vi "IX83 Send Command.vi"(0 "Connection ID":refnum<k5>, 2 "Wait for Reply":bool=TRUE, 7 "Cmd":string, 11 "Error In":errorcluster) -> (4 "Connection ID Out":refnum<k5>, 8 "CMD Reply":string, 15 "Error Out":errorcluster)   [LabVIEW 2020]
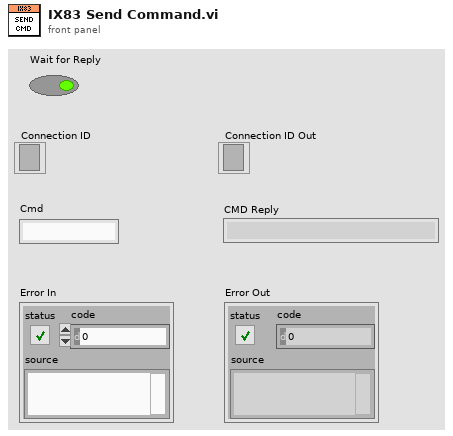
[diagram p1: front panel]
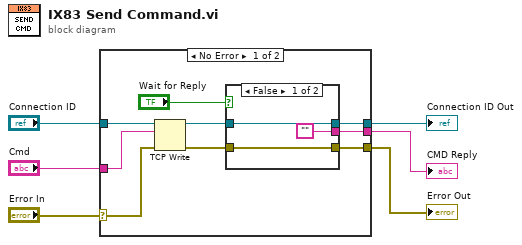
[diagram p0: block diagram]
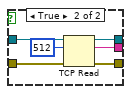
[diagram p2: hidden frame]
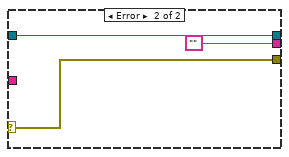
[diagram p3: hidden frame]
diagram:
  n1 = case shown="No Error" "Error In" {
    selector: "Error In" -> [w11 w27]
    tunnel: "Connection ID" -> [w13 w26]
    tunnel: [w12 w26] -> w5
    tunnel: [w10 ""] -> w3
    tunnel: [w9 w27] -> w2
    tunnel: "Cmd" -> [w8 _]
    frame No Error {
      n2 = TCP Write(connection ID=w13, data in=w8, error in (no error)=w11) -> (connection ID out=w15:refnum<k5>, error out=w14:errorcluster)  [unwired: 1 in, 1 out]
      n3 = case shown="False" "Wait for Reply" {
        tunnel: w15 -> [w18 w24]
        tunnel: w14 -> [w17 w23]
        tunnel: [w18 w21] -> w12
        tunnel: ["" w20] -> w10
        tunnel: [w17 w19] -> w9
        frame False {
        }
        frame True {
          n4 = TCP Read(connection ID=w24, bytes to read=512, error in (no error)=w23) -> (connection ID out=w21:refnum<k5>, data out=w20:string, error out=w19:errorcluster)  [unwired: 2 in]
        }
      }
    }
    frame Error {
    }
  }
  "CMD Reply" <- w3
  "Connection ID Out" <- w5
  "Error Out" <- w2
